vi "test setting.vi"() -> ()   [LabVIEW 2013]
uses:
  lightfield-automation-labview/VIs/ClientServerMode/CS_LFAClassGlobal.vi
  lightfield-automation-labview/LightField Automation.lvclass
panel:
  in  "ADC Quality":u16(ring) items=["ElectronMultiplied"=3, "LowNoise"=1]
  out "Array":variant[](array[variant])
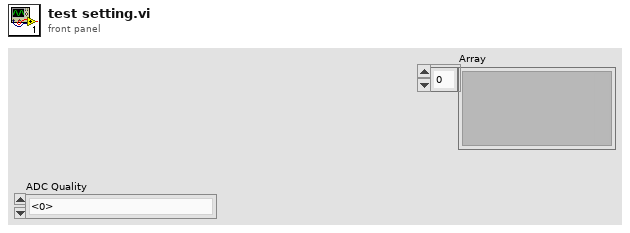
[diagram p1: front panel]
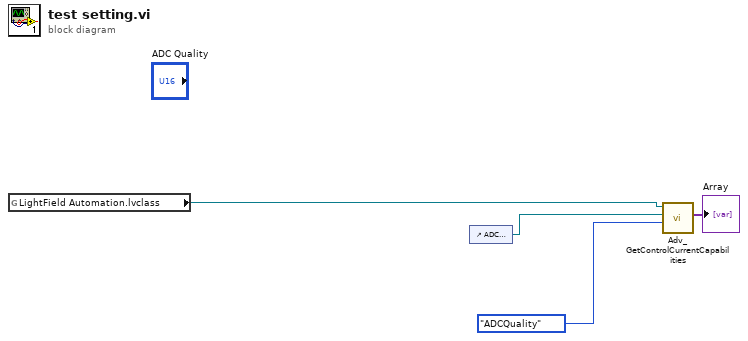
[diagram p0: block diagram]
diagram:
  n1 = global read "CS_LFAClassGlobal.vi" "LightField Automation.lvclass"() -> (w4:refnum<class "LightField Automation.lvclass">)
  n2 = control-ref of="ADC Quality"() -> (w2:refnum<vi>)
  n3 = call "Adv_GetControlCurrentCapabilities.vi"("Setting"=enum16{"ADCGain", "ADCQuality"}."ADCQuality", "Control"=w2, "LightField Automation in"=w4) -> ("Array"=→"Array":variant[])  [unwired: 6 in, 2 out]
